vi "eventSettingVersions.vi"(8 "error in (no error)":errorcluster, 11 "Publisher in":refnum<class "Publisher.lvclass">) -> (0 "error out":errorcluster, 3 "Publisher out":refnum<class "Publisher.lvclass">)   [LabVIEW 2016, in "Publisher.lvclass"]
uses:
  Publisher.lvclass
  Publisher.lvclass/Publisher.ctl
  Communicator/Communicator/Communicator.lvclass
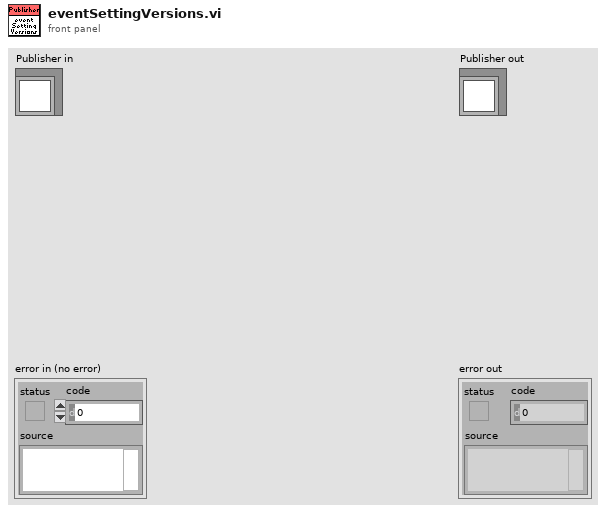
[diagram p1: front panel]
types:
  T1 = typedef "M1M3SupportTopics.lvlib/EventSettingVersions.ctl" = cluster{"Timestamp":T2, "RecommendedSettingsVersion":string}
  T2 = typedef "M1M3SupportTopics.lvlib/Timestamp.ctl" = dbl
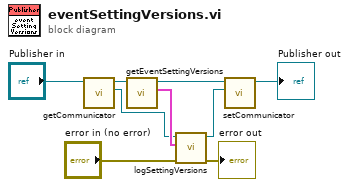
[diagram p0: block diagram]
diagram:
  n1 = call "getCommunicator.vi"("Publisher in"="Publisher in") -> ("Communicator"=w5:refnum<class "Communicator.lvclass">, "Publisher out"=w7:refnum<class "Publisher.lvclass">)  [unwired: 9 in]
  n2 = call "getEventSettingVersions.vi"("Publisher in"=w7) -> ("EventSettingVersions"=w6:T1, "Publisher out"=w3:refnum<class "Publisher.lvclass">)  [unwired: 9 in]
  n3 = call-dynamic "logSettingVersions.vi"("error in (no error)"="error in (no error)", "EventSettingVersions"=w6, "Communicator in"=w5) -> ("error out"=→"error out":errorcluster, "Communicator out"=w4:refnum<class "Communicator.lvclass">)  [unwired: 7 in]
  n4 = call "setCommunicator.vi"("Communicator"=w4, "Publisher in"=w3) -> ("Publisher out"=→"Publisher out":refnum<class "Publisher.lvclass">)  [unwired: 9 in]
